vi "Problem1.1.vi"() -> ()   [LabVIEW 2018]
panel:
  in  "?":bool
  in  "B":bool
  out "Not B":bool
  out "Not A":bool
  out "XOR":bool
  out "Or":bool
  out "And":bool
  in  "A":bool
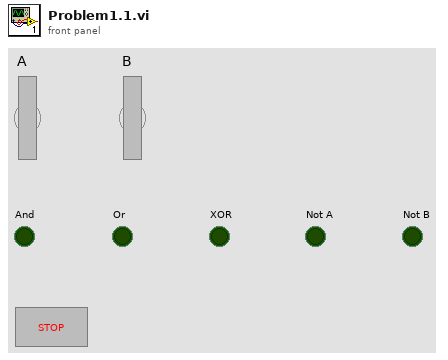
[diagram p1: front panel]
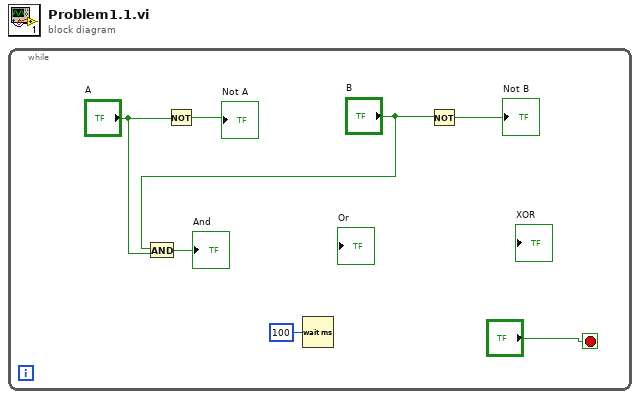
[diagram p0: block diagram]
diagram:
  n1 = while {
    stop <- "?" stop-if-true
    n2 = And(x="B", y="A") -> (x .and. y?=→"And":bool)
    n3 = Not(x="A") -> (.not. x?=→"Not A":bool)
    n4 = Wait (ms)(milliseconds to wait=u32 100) -> ()  [unwired: 1 out]
    n5 = Not(x="B") -> (.not. x?=→"Not B":bool)
  }
